vi "Safety XOR by name.vi"(8 "error in (no error)":errorcluster, 9 "Target Digital in":u32, 10 "Value to Write":bool, 11 "DIG_IO in":refnum<class "DIG_IO.lvclass">) -> (0 "error out":errorcluster, 1 "Value Select":bool, 2 "Target Digital out":u32, 3 "DIG_IO out":refnum<class "DIG_IO.lvclass">)   [LabVIEW 2019, in "DIG_IO.lvlib" / "DIG_IO.lvclass"]
uses:
  Library/DIG_IO.lvclass
  Library/DIG_IO.lvclass/DIG_IO.ctl
  Accessors/Read Digital.vi
  Accessors/Read Channel Names.vi
  Accessors/Read XOR List.vi
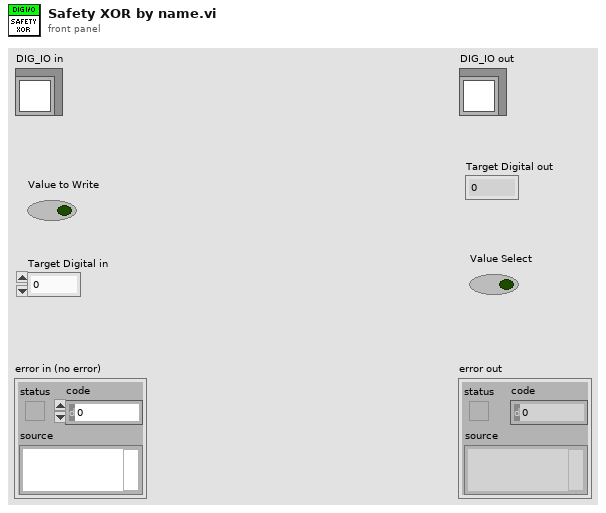
[diagram p1: front panel]
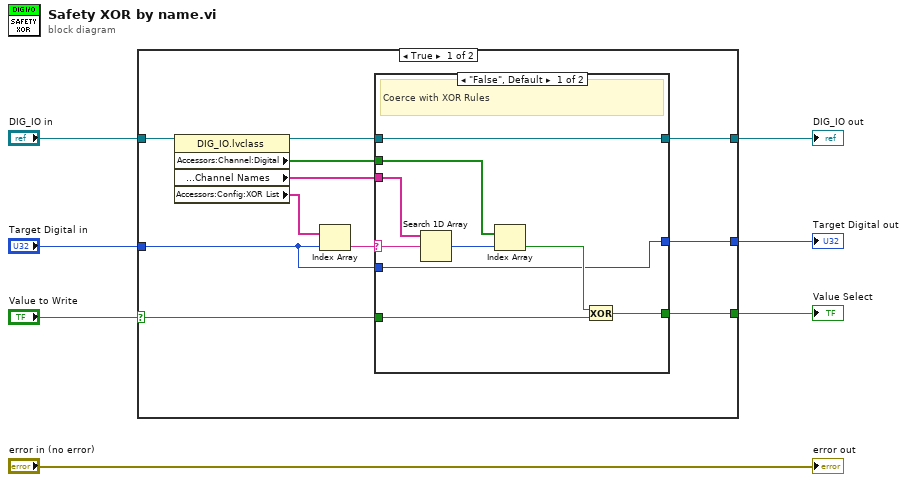
[diagram p0: block diagram]
diagram:
  n1 = case shown="True" "Value to Write" {
    selector: "Value to Write" -> [w8 w31]
    tunnel: [w14 w33] -> w6
    tunnel: "DIG_IO in" -> [w18 w33]
    tunnel: "Target Digital in" -> [w10 w32]
    tunnel: [w12 w31] -> w4
    tunnel: [w9 w32] -> w3
    frame True {
      n2 = property class="DIG_IO.lvclass"(reference=w18) -> (reference out=w15:refnum<class "DIG_IO.lvclass">, "Accessors:Channel:Digital"=w11:bool[], "Accessors:Channel:Channel Names"=w13:string[], "Accessors:Config:XOR List"=w17:string[])  [unwired: 1 in, 1 out]
      n3 = Index Array(array=w17, index=w10) -> (element=w16:string)
      n4 = case shown="\"False\", Default" w16 {
        selector: w16 -> [w26 _]
        tunnel: w15 -> [w20 w30]
        tunnel: [w20 w30] -> w14
        tunnel: w13 -> [w27 _]
        tunnel: w8 -> [w22 w29]
        tunnel: [w21 w29] -> w12
        tunnel: w11 -> [w25 _]
        tunnel: w10 -> [w19 w28]
        tunnel: [w19 w28] -> w9
        frame "False", Default {
          # "Coerce with XOR Rules"
          n5 = Search 1D Array(1D array=w27, element=w26) -> (index of element=w24:i32)  [unwired: 1 in]
          n6 = Index Array(array=w25, index=w24) -> (element=w23:bool)
          n7 = Exclusive Or(1:w22, 2:w23) -> (0:w21:bool)
        }
        frame "" {
          # "Empty String implies there is no XOR Requirement"
        }
      }
    }
    frame False {
    }
  }
  "DIG_IO out" <- w6
  "Value Select" <- w4
  "Target Digital out" <- w3
  "error out" <- "error in (no error)"
